vi "move one step(angle command in degree).vi"(6 "ID":i16[](array[numeric])=[1, 2, 3, 4], 7 "theta4a":dbl, 8 "theta3a":dbl, 9 "theta2a":dbl, 10 "theta1a":dbl) -> ()   [LabVIEW 2017]
panel:
  out "function return":i32
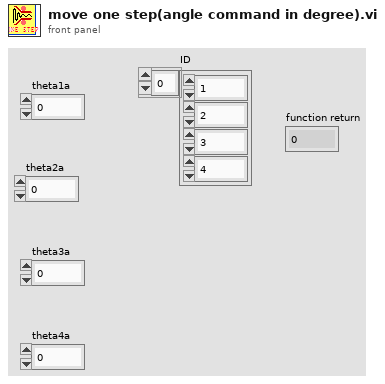
[diagram p1: front panel]
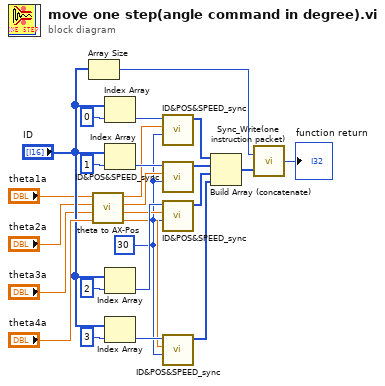
[diagram p0: block diagram]
diagram:
  w11 = 30
  n1 = Array Size(array="ID") -> (size(s)=w10:i32)
  n2 = call "theta to AX-Pos.vi"("theta4a"="theta4a", "theta3a"="theta3a", "theta2a"="theta2a", "theta1a"="theta1a") -> ("DEG 4"=w12:dbl, "DEG 3"=w13:dbl, "DEG 2"=w14:dbl, "DEG1"=w15:dbl)
  n3 = Index Array(array="ID", index=0) -> (element=w19:i16)
  n4 = Index Array(array="ID", index=1) -> (element=w18:i16)
  n5 = Index Array(array="ID", index=2) -> (element=w17:i16)
  n6 = Index Array(array="ID", index=3) -> (element=w16:i16)
  n7 = call "ID&POS&SPEED_sync.vi"("speed"=w11, "Ax-Pos"=w15, "ID"=w19) -> ("ID&POS&SPEED"=w9:u8[])  [unwired: 8 in]
  n8 = call "ID&POS&SPEED_sync.vi"("speed"=w11, "Ax-Pos"=w14, "ID"=w18) -> ("ID&POS&SPEED"=w8:u8[])  [unwired: 8 in]
  n9 = call "ID&POS&SPEED_sync.vi"("speed"=w11, "Ax-Pos"=w13, "ID"=w17) -> ("ID&POS&SPEED"=w7:u8[])  [unwired: 8 in]
  n10 = call "ID&POS&SPEED_sync.vi"("speed"=w11, "Ax-Pos"=w12, "ID"=w16) -> ("ID&POS&SPEED"=w6:u8[])  [unwired: 8 in]
  n11 = Build Array (concatenate)(w9, w8, w7, w6) -> (w5:u8[])
  n12 = call "Sync_Write(one instruction packet).vi"("ID&DEG_code&\nSpeed_code"=w5, "Actuator Number"=w10) -> ("function return"=→"function return":i32)
